vi "PC_Pub_imgFile setSessionNum.vi"(8 "error in (no error)":errorcluster, 10 "newSessionString":string, 11 "imgFile in":refnum<class "PC_Pub_imgFile.lvclass">) -> (0 "error out":errorcluster, 3 "imgFile out":refnum<class "PC_Pub_imgFile.lvclass">)   [LabVIEW 2018, in "PC_Pub_imgFile.lvclass"]
uses:
  PC_Pub_imgFile.lvclass
  PC_Pub_imgFile.lvclass/PC_Pub_imgFile.ctl
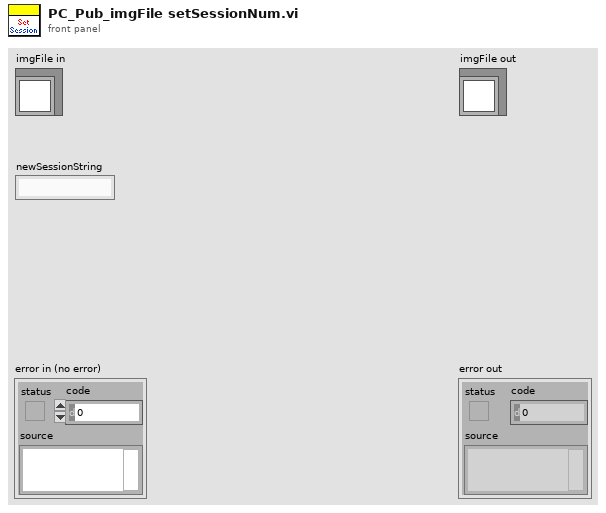
[diagram p1: front panel]
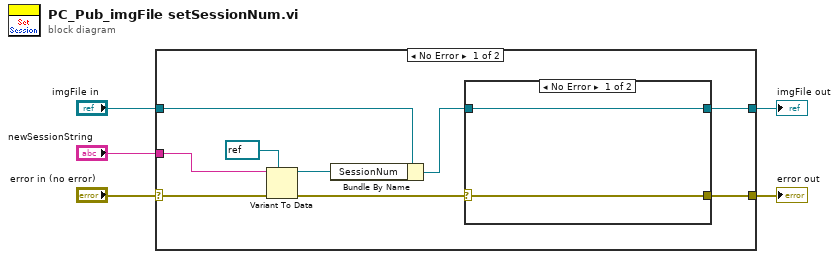
[diagram p0: block diagram]
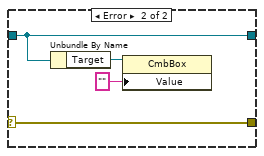
[diagram p2: hidden frame]
diagram:
  n1 = case shown="No Error" "error in (no error)" {
    selector: "error in (no error)" -> [w12 w22]
    tunnel: [w7 w22] -> w4
    tunnel: [w6 w21] -> w2
    tunnel: "imgFile in" -> [w11 w21]
    tunnel: "newSessionString" -> [w13 _]
    frame No Error {
      n2 = Variant To Data(error in=w12, type=refnum<k21> refnum ("SessionNum"), Variant=w13) -> (data=w10:refnum<k21>, error out=w8:errorcluster)
      n3 = Bundle By Name(cluster=w11, "SessionNum"=w10) -> (w9:refnum<class "PC_Pub_imgFile.lvclass">)
      n4 = case shown="No Error" w8 {
        selector: w8 -> [w15 w18]
        tunnel: w9 -> [w16 w17]
        tunnel: [w15 w18] -> w7
        tunnel: [w16 w17] -> w6
        frame No Error {
        }
        frame Error {
          n5 = Unbundle By Name(w17) -> ("Target"=w20:refnum<vi>)
          n6 = property class="CmbBox"(reference=w20, "Value"="") -> ()  [unwired: 1 in, 2 out]
        }
      }
    }
    frame Error {
    }
  }
  "error out" <- w4
  "imgFile out" <- w2
